vi "P116x1ch_ComandoSecuencia.vi"(8 "Dwell Time(min)":T1, 9 "Rate(C/min)":T1, 10 "Setpoint(C)":T1) -> (0 "Dwell Time(min) 2":T1, 1 "Rate(C/min) 2":T1, 2 "Setpoint(C) 2":T1, 3 "Cancel 2":bool)   [LabVIEW 2017]
uses:
  1xP116.ctl
panel:
  in  "Cancel":bool
  in  "Write":bool
  # "Eurotherm"
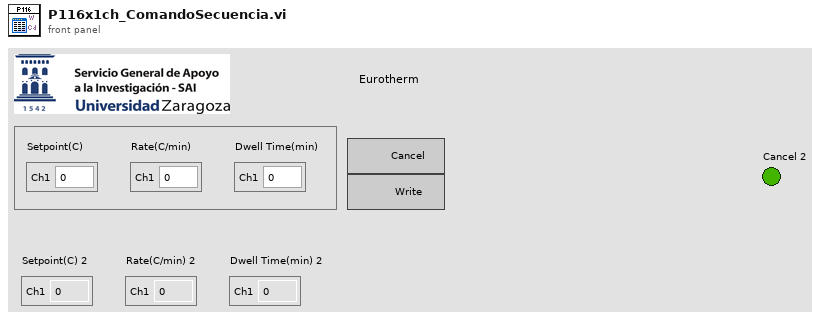
[diagram p1: front panel]
types:
  T1 = typedef "1xP116.ctl" = cluster{"Ch1":dbl}
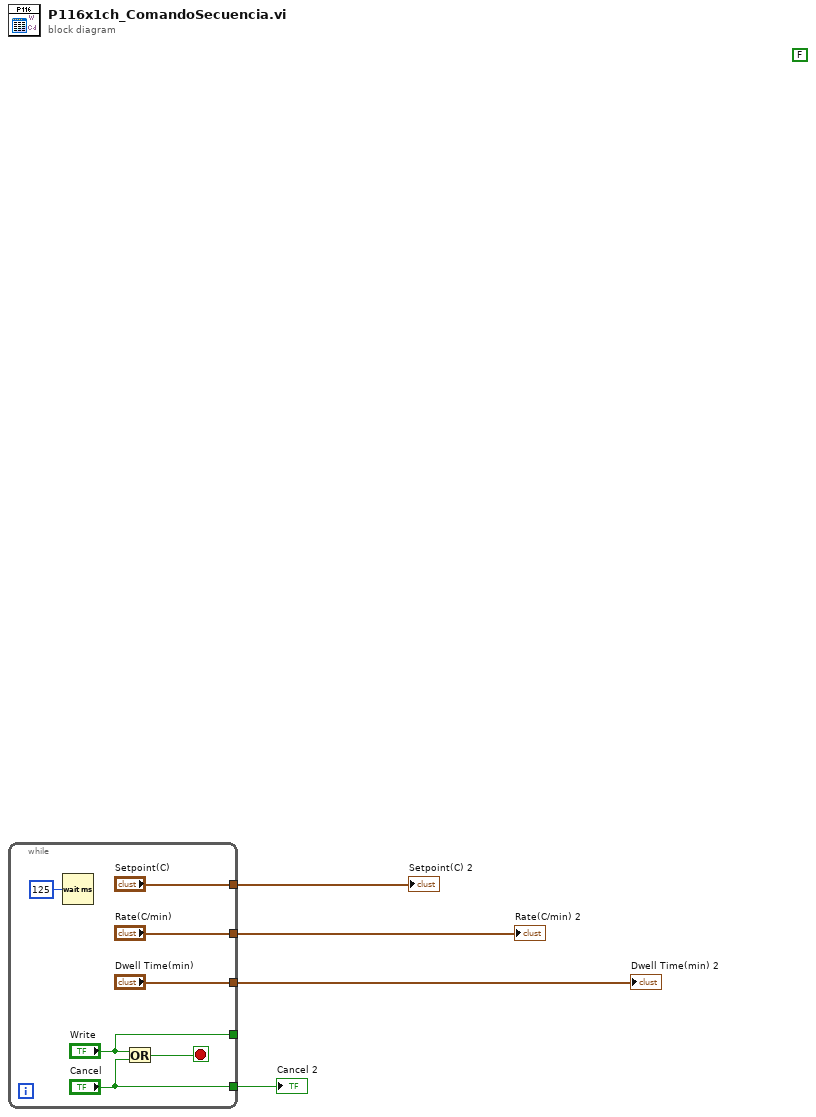
[diagram p0: block diagram]
diagram:
  (unwired) FALSE
  n1 = while {
    tunnel: ["Cancel"] -> w4
    tunnel: ["Setpoint(C)"] -> w3
    tunnel: ["Rate(C/min)"] -> w2
    tunnel: ["Write"] -> _
    tunnel: ["Dwell Time(min)"] -> w1
    stop <- w6 stop-if-true
    n2 = Wait (ms)(milliseconds to wait=u32 125) -> ()  [unwired: 1 out]
    n3 = Or(x="Write", y="Cancel") -> (x .or. y?=w6:bool)
  }
  "Cancel 2" <- w4
  "Setpoint(C) 2" <- w3
  "Rate(C/min) 2" <- w2
  "Dwell Time(min) 2" <- w1
